vi "Joysticks Active.vi"() -> (0 "Secondary Controller Buttons":T1, 1 "Secondary Controller Axes":T2, 2 "Primary Controller Buttons":T1, 3 "Primary Controller Axes":T2)   [LabVIEW 2012]
uses:
  <vilib>/Rock Robotics/WPI/Joystick/WPI_JoystickButtonState.ctl
  <vilib>/Rock Robotics/WPI/Joystick/WPI_JoystickGetSetRefNum.vi
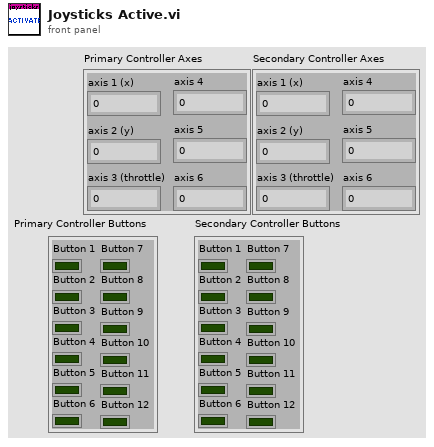
[diagram p1: front panel]
types:
  T1 = typedef "WPI_JoystickButtonState.ctl" = cluster{"Button 1":bool, "Button 2":bool, "Button 3":bool, "Button 4":bool, "Button 5":bool, "Button 6":bool, "Button 7":bool, "Button 8":bool, "Button 9":bool, "Button 10":bool, "Button 11":bool, "Button 12":bool}
  T2 = cluster{"axis 1 (x)":dbl, "axis 2 (y)":dbl, "axis 3 (throttle)":dbl, "axis 4":dbl, "axis 5":dbl, "axis 6":dbl}
  T3 = typedef "WPI_JoystickDevRef.ctl" = cluster{"Device":T4}
  T4 = typedef "WPI_JoystickDeviceEnum.ctl" = enum16{"USB 1", "USB 2", "USB 3", "USB 4", "Kinect 1", "Kinect 2"}
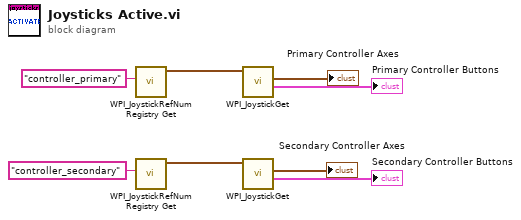
[diagram p0: block diagram]
diagram:
  n1 = call <vilib>:"WPI_JoystickRefNum Registry Get.vi"("refnum name"="controller_primary") -> ("JoystickDevRef"=w8:T3)  [unwired: 9 in, 1 out]
  n2 = call <vilib>:"WPI_JoystickRefNum Registry Get.vi"("refnum name"="controller_secondary") -> ("JoystickDevRef"=w5:T3)  [unwired: 9 in, 1 out]
  n3 = call <vilib>:"WPI_JoystickGet.vi"("JoystickDevRef"=w8) -> ("Buttons"=→"Primary Controller Buttons":T1, "Axes"=→"Primary Controller Axes":T2)  [unwired: 4 in, 1 out]
  n4 = call <vilib>:"WPI_JoystickGet.vi"("JoystickDevRef"=w5) -> ("Buttons"=→"Secondary Controller Buttons":T1, "Axes"=→"Secondary Controller Axes":T2)  [unwired: 4 in, 1 out]
